vi "_Create ISO 8601 File Name.vi"(7 "Start Time Stamp":timestamp, 8 "Error In":errorcluster, 11 "Log Folder":path) -> (0 "Error Out":errorcluster, 3 "ISO 8601 File":path)   [LabVIEW 2014, in "CF-Logger.lvlib"]
uses:
  CF-Logger.lvlib
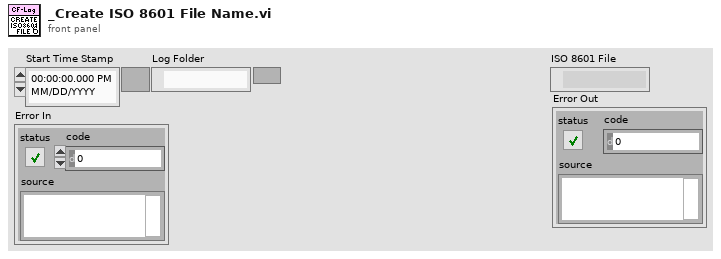
[diagram p1: front panel]
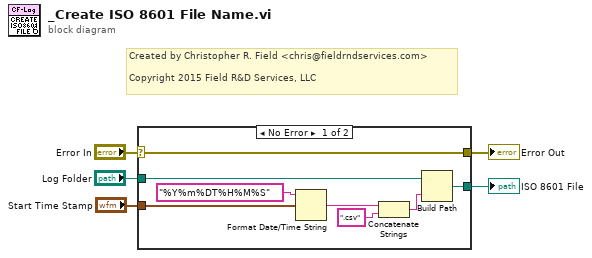
[diagram p0: block diagram]
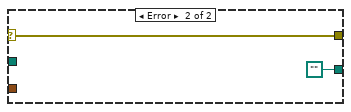
[diagram p2: hidden frame]
diagram:
  # "Created by Christopher R. Field <chris@fieldrndservices.com>\n\nCopyright 2015 Field R&D Services, LLC"
  n1 = case shown="No Error" "Error In" {
    selector: "Error In" -> [w6 w15]
    tunnel: "Start Time Stamp" -> [w9 _]
    tunnel: "Log Folder" -> [w8 _]
    tunnel: [w7 path ""] -> w2
    tunnel: [w6 w15] -> w1
    frame No Error {
      n2 = Format Date/Time String(time format string (%c)="%Y%m%DT%H%M%S", seconds (now)=w9) -> (date/time string=w12:string)  [unwired: 1 in]
      n3 = Concatenate Strings(w12, ".csv" ("string")) -> (w10:string)
      n4 = Build Path(base path=w8, name or relative path=w10) -> (appended path=w7:path)
    }
    frame Error {
    }
  }
  "ISO 8601 File" <- w2
  "Error Out" <- w1
